vi "Get Model Roll Pitch Yaw.vi"(0 "Traverse Name":string, 1 "Mode":T2) -> (2 "Model:    Roll        Pitch         Yaw  (deg)":sgl[](array[numeric]) caption="ModelRollPitchYaw (deg)" format="%#.2f", 3 "Position Feedback System":T1, 4 "Error String":string)   [LabVIEW 2021]
uses:
  Controls/User_Specific_mode.ctl
  ADAM Client/Sub VIs/ADAM Controls/Quick_local_ADAM_Table.ctl
  Controls/Position Feedback System.ctl
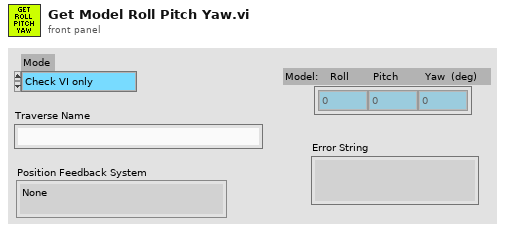
[diagram p1: front panel]
types:
  T1 = typedef "Position Feedback System.ctl" = enum16{"None", "OptiTrack"}
  T2 = typedef "User_Specific_mode.ctl" = enum16{"Check VI only", "Run VI"}
  T3 = typedef "Quick_local_ADAM_Table.ctl" = enum16{"Read Global", "Load Global From ADAM Table", "Write Global"}
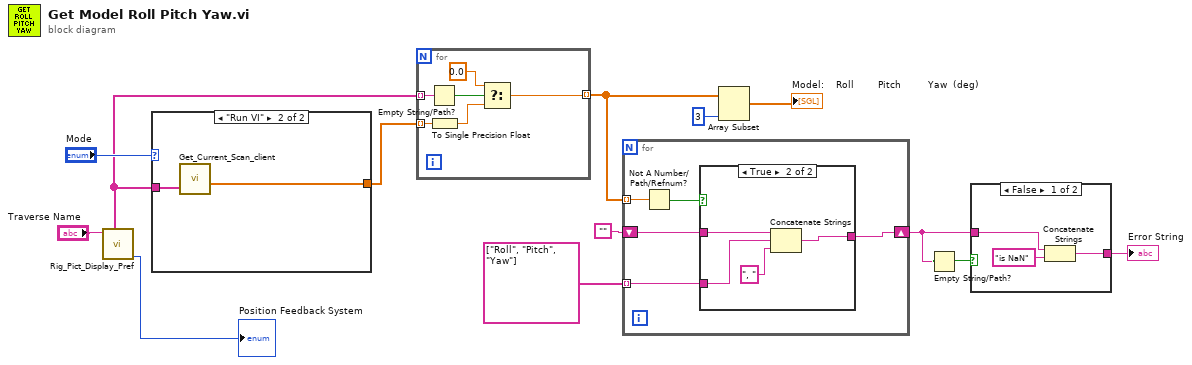
[diagram p0: block diagram]
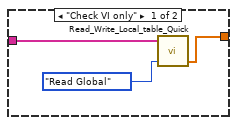
[diagram p4: hidden frame]
diagram:
  n1 = call "Rig_Pict_Display_Pref.vi"("Traverse Name"="Traverse Name") -> ("Roll Pitch Yaw ADAM Channels"=w2:string[], "Position Feedback System"=→"Position Feedback System":T1)  [unwired: 2 in, 4 out]
  n2 = case shown="\"Run VI\"" "Mode" {
    tunnel: [w15 w17] -> w4
    tunnel: w2 -> [w16 w18]
    frame "Check VI only" {
      n3 = call "Read_Write_Local_table_Quick.vi"("Mode"=Quick_local_ADAM_Table."Read Global", "Ch names In"=w16) -> ("Numeric Values Out"=w15:dbl[])  [unwired: 1 in, 2 out]
    }
    frame "Run VI" {
      n4 = call "Get_Current_Scan_client.vi"("multipleChannels"=w18) -> ("Numerical Values"=w17:dbl[])  [unwired: 1 in, 3 out]
    }
  }
  n5 = for {
    tunnel: w2 -> [w24] mode=indexing
    tunnel: w4 -> [w22] mode=indexing
    tunnel: [w20] -> w3 mode=indexing
    n6 = Empty String/Path?(string/path=w24) -> (empty?=w23:bool)
    n7 = To Single Precision Float(number=w22) -> (single precision float=w19:sgl)
    n8 = Select(t=sgl 0.0, s=w23, f=w19) -> (s? t:f=w20:sgl)
  }
  n9 = for {
    tunnel: w3 -> [w29] mode=indexing
    shift-right: [w25] -> w5
    shift-left: "" -> [w27]
    tunnel: string[] ["Roll", "Pitch", "Yaw"] ("appended array") -> [w26] mode=indexing
    n10 = Not A Number/Path/Refnum?(number/path/refnum=w29) -> (NaN/Path/Refnum?=w28:bool)
    n11 = case shown="True" w28 {
      tunnel: w27 -> [w30 w34]
      tunnel: w26 -> [_ w33]
      tunnel: [w30 w32] -> w25
      frame False {
      }
      frame True {
        n12 = Concatenate Strings(w34, w33, ", " ("string")) -> (w32:string)
      }
    }
  }
  n13 = Array Subset(array=w3, length=3) -> (→"Model:    Roll        Pitch         Yaw  (deg)":sgl[])  [unwired: 1 in]
  n14 = Empty String/Path?(string/path=w5) -> (empty?=w7:bool)
  n15 = case shown="False" w7 {
    tunnel: [w35 w38] -> w6
    tunnel: w5 -> [w37 w38]
    frame False {
      n16 = Concatenate Strings(w37, "is NaN" ("string")) -> (w35:string)
    }
    frame True {
    }
  }
  "Error String" <- w6
